vi "Check Missed Samples.vi"(8 "error in (no error)":errorcluster, 11 "Waveform Receive in":refnum<class "Waveform Receive.lvclass">) -> (0 "error out":errorcluster, 1 "Samples Missed":u64, 2 "Missing Samples?":bool, 3 "Waveform Receive out":refnum<class "Waveform Receive.lvclass">)   [LabVIEW 2015, in "Waveform Receive.lvclass"]
uses:
  Waveform Receive.lvclass
  Waveform Receive.lvclass/Waveform Receive.ctl
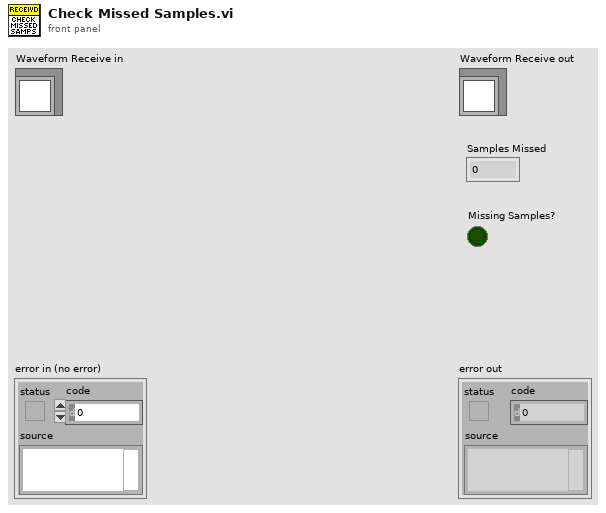
[diagram p1: front panel]
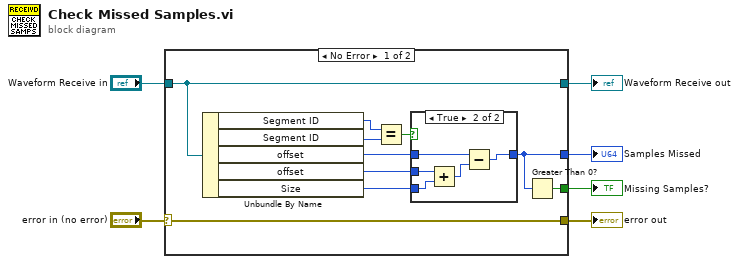
[diagram p0: block diagram]
diagram:
  n1 = case shown="No Error" "error in (no error)" {
    selector: "error in (no error)" -> [w16 w24]
    tunnel: [w16 w24] -> w5
    tunnel: [w12 w23] -> w3
    tunnel: "Waveform Receive in" -> [w12 w23]
    tunnel: [w7 _] -> w2
    tunnel: [w8 _] -> w1
    frame No Error {
      n2 = Unbundle By Name(w12) -> ("Segment ID"=w10:u64, "Segment ID"=w11:u64, "offset"=w13:u64, "offset"=w15:u64, "Size"=w14:i32)
      n3 = Equal?(x=w10, y=w11) -> (x = y?=w9:bool)
      n4 = case shown="True" w9 {
        tunnel: [w17 w22] -> w7
        tunnel: w15 -> [_ w21]
        tunnel: w14 -> [_ w20]
        tunnel: w13 -> [w17 w19]
        frame False {
        }
        frame True {
          n5 = Add(x=w21, y=w20) -> (x+y=w18:u64)
          n6 = Subtract(x=w19, y=w18) -> (x-y=w22:u64)
        }
      }
      n7 = Greater Than 0?(x=w7) -> (x > 0?=w8:bool)
    }
    frame Error {
    }
  }
  "error out" <- w5
  "Waveform Receive out" <- w3
  "Missing Samples?" <- w1
  "Samples Missed" <- w2
